vi "Configure Module.vi"(8 "error in (no error)":errorcluster, 10 "IOV ref in":variant, 11 "Module Template in":refnum<class "9207.lvclass">) -> (0 "error out":errorcluster, 2 "IOV ref out":variant, 3 "Module Template out":refnum<class "9207.lvclass">)   [LabVIEW 2017, in "Modules.lvlib" / "9207.lvclass"]
uses:
  9207.lvclass
  <resource>/objmgr/cRIO.rc
  RSI Module/RSI Module.lvclass
  C:/Users/nitest/Desktop/Git 2017/niveristand-scan-engine-module-libraries/Source/RSI Module/RSI Module.lvclass
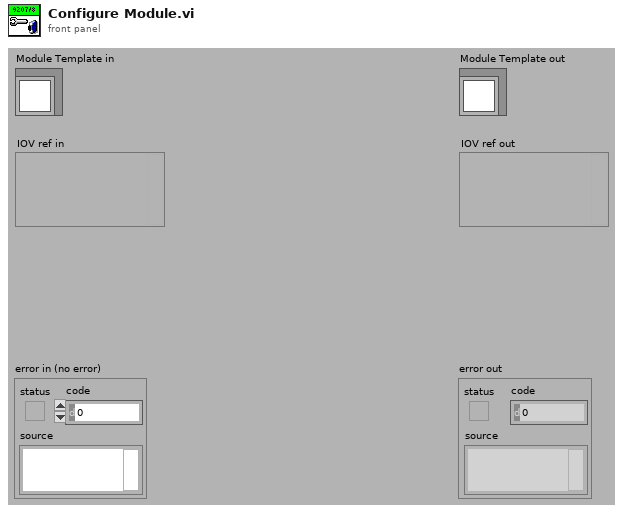
[diagram p1: front panel]
types:
  T1 = typedef "Modules.lvlib/RSI Module.lvclass/Module Models.ctl" = enum16{"Empty", "NI 9201", "NI 9203", "NI 9205", "NI 9206", "NI 9207", "NI 9208", "NI 9209", "NI 9210", "NI 9211", "NI 9212", "NI 9213", "NI 9214", "NI 9215", "NI 9216", "NI 9217", "NI 9219", "NI 9220", "NI 9221", "NI 9222", "NI 9223", "NI 9224", "NI 9225", "NI 9226", "NI 9227", "NI 9228", "NI 9229", "NI 9233", "NI 9234", "NI 9235", "NI 9236", "NI 9237", "NI 9239", "NI 9242", "NI 9244", "NI 9253", "NI 9263", "NI 9264", "NI 9265", "NI 9266", "NI 9269", "NI 9344", "NI 9350", "NI 9375", "NI 9401", "NI 9402", "NI 9403", "NI 9411", "NI 9421", "NI 9422", "NI 9423", "NI 9425", "NI 9426", "NI 9435", "NI 9436", "NI 9437", "NI 9472", "NI 9474", "NI 9475", "NI 9476", "NI 9477", "NI 9478", "NI 9481", "NI 9482", "NI 9485"}
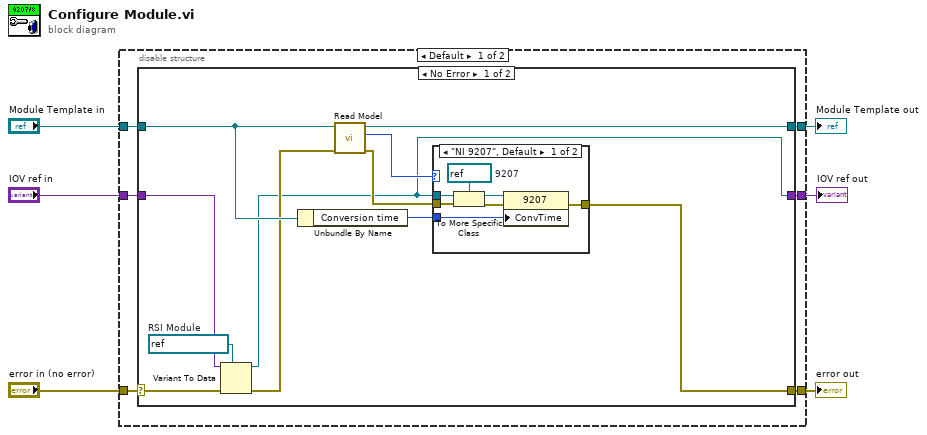
[diagram p0: block diagram]
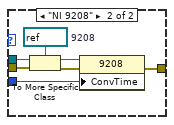
[diagram p2: hidden frame]
diagram:
  n1 = disable-structure shown="Default" {
    disable-tunnel: "error in (no error)" -> [w12 w41]
    disable-tunnel: [w11 w41] -> w5
    disable-tunnel: "Module Template in" -> [w10 w43]
    disable-tunnel: [w9 w43] -> w3
    disable-tunnel: "IOV ref in" -> [w8 w42]
    disable-tunnel: [w7 w42] -> w1
    frame condition #0 (active) {
      n2 = case shown="No Error" w12 {
        selector: w12 -> [w19 w40]
        tunnel: [w23 w40] -> w11
        tunnel: [w20 w39] -> w9
        tunnel: w10 -> [w21 w39]
        tunnel: w8 -> [w15 w38]
        tunnel: [w14 w38] -> w7
        frame No Error {
          w13 = refnum<k21> refnum  # RSI Module
          n3 = Variant To Data(error in=w19, type=w13, Variant=w15) -> (data=w14:refnum<k21>, error out=w16:errorcluster)
          n4 = Unbundle By Name(w21) -> ("Conversion time"=w22:u32)
          n5 = call "Read Model.vi"("error in (no error)"=w16, "RSI Module in"=w21) -> ("error out"=w18:errorcluster, "Model"=w17:T1, "RSI Module out"=w20:refnum<class "9207.lvclass">)  [unwired: 7 in]
          n6 = case shown="\"NI 9207\", Default" w17 {
            tunnel: w18 -> [w30 w37]
            tunnel: [w26 w33] -> w23
            tunnel: w14 -> [w25 w32]
            tunnel: w22 -> [w24 w31]
            frame "NI 9207", Default {
              w29 = refnum<k21> refnum  # 9207
              n7 = To More Specific Class(target class=w29, reference=w25, error in=w30) -> (specific class reference=w28:refnum<k21>, error out=w27:errorcluster)
              n8 = property class="9207"(reference=w28, error in=w27, "ConvTime"=w24) -> (error out=w26:errorcluster)  [unwired: 1 out]
            }
            frame "NI 9208" {
              w36 = refnum<k21> refnum  # 9208
              n9 = To More Specific Class(target class=w36, reference=w32, error in=w37) -> (specific class reference=w35:refnum<k21>, error out=w34:errorcluster)
              n10 = property class="9208"(reference=w35, error in=w34, "ConvTime"=w31) -> (error out=w33:errorcluster)  [unwired: 1 out]
            }
          }
        }
        frame Error {
        }
      }
    }
    frame condition #1 {
    }
  }
  "error out" <- w5
  "Module Template out" <- w3
  "IOV ref out" <- w1
